vi "test Script CD with Configuration.vi"(8 "error in":errorcluster, 11 "TestCase in":refnum<class "Scripting.lvclass">) -> (0 "error out":errorcluster, 3 "TestCase out":refnum<class "Scripting.lvclass">)   [LabVIEW 2020, in "Scripting.lvclass"]
uses:
  Scripting.lvclass
  C:/Git/niveristand-custom-device-testing-tools/VeriStandScriptingTestCase/VeriStandScriptingTestCase.lvclass
  Shared/1553 Channel.ctl
  Shared/Address.ctl
  Shared/Message Definition.ctl
  Shared/Message Type.ctl
  Shared/Terminal Endpoint.ctl
  Shared/Parameter Definition.ctl
  niveristand-custom-device-testing-tools/VeriStandScriptingTestCase/VeriStandScriptingTestCase.lvclass/VeriStandScriptingTestCase.ctl
  niveristand-custom-device-testing-tools/VeriStandScriptingTestCase/Read Target.vi
  NationalInstruments.VeriStand.SystemDefinitionAPI
  <vilib>/addons/_JKI Toolkits/VI Tester/TestCase.llb/TestCase.lvclass
  Scripting/Ballard MIL-STD-1553 Scripting.lvlib
  C:/Program Files (x86)/National Instruments/LabVIEW 2020/vi.lib/addons/_JKI Toolkits/VI Tester/TestCase.llb/TestCase.lvclass
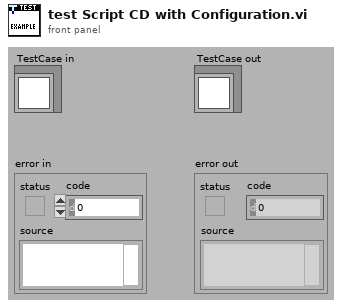
[diagram p1: front panel]
types:
  T1 = typedef "1553 Channel.ctl" = cluster{"HW channel":u16, "terminal addresses":T2[], "acyclic frame names":string[], "messages":T3[]}
  T2 = typedef "Address.ctl" = u16
  T3 = typedef "Message Definition.ctl" = cluster{"name":string, "message type":T4, "endpoint Tx":T5, "endpoint Rx":T5, "create timestamp channel":bool, "mode code":u16, "number of words":u16, "parameters":cluster{"name":string, "default value":dbl, "unit":string, "parameter definition":T6}[]}
  T4 = typedef "Message Type.ctl" = string
  T5 = typedef "Terminal Endpoint.ctl" = cluster{"terminal address":T2, "subaddress":T2}
  T6 = typedef "Parameter Definition.ctl" = cluster{"start index":i32, "size (bits)":i32, "encoding":enum16{"BNR", "BCD", "Discrete"}, "signed":bool, "multiplier":dbl, "offset":dbl}
  T7 = typedef "Custom Device API.lvlib/Custom Device Item Ref.ctl" = u64
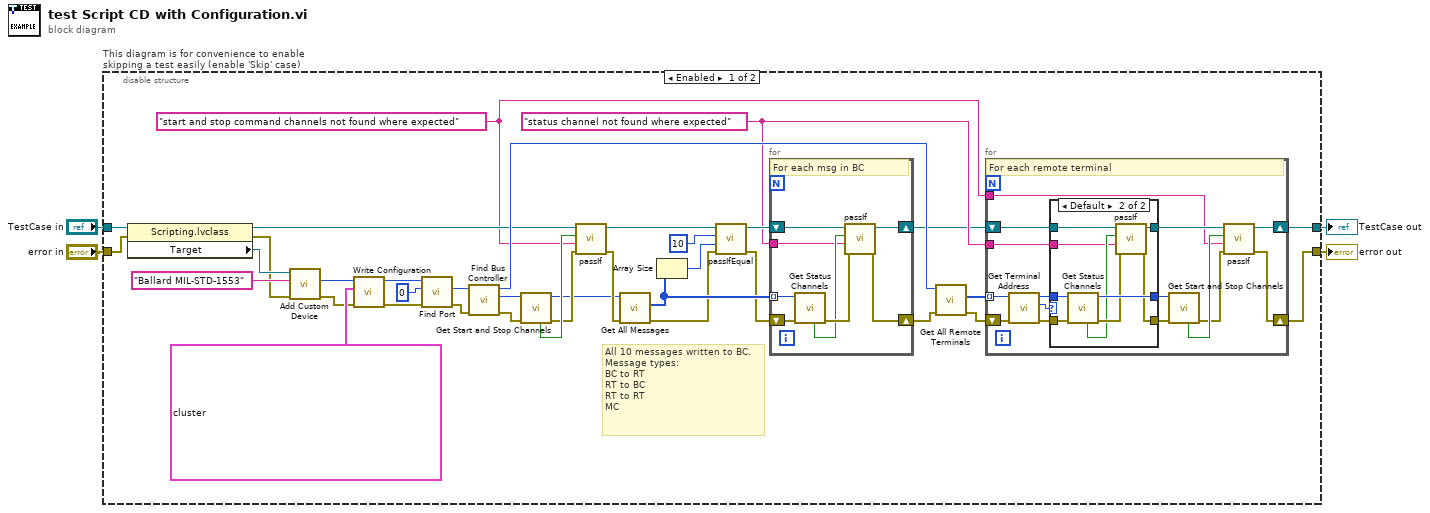
[diagram p0: block diagram]
diagram:
  n1 = disable-structure "This diagram is for convenience to enable skipping a test easily (enable 'Skip' case)" shown="Enabled" {
    disable-tunnel: "TestCase in" -> [w39 w79]
    disable-tunnel: [w22 w77] -> w1
    disable-tunnel: [w21 w78] -> w3
    disable-tunnel: "error in" -> [w34 w76]
    frame Enabled {
      w7 = "start and stop command channels not found where expected" ("name")
      w15 = "status channel not found where expected" ("name")
      # "All 10 messages written to BC.\nMessage types:\nBC to RT\nRT to BC\nRT to RT\nMC"
      n2 = property class="Scripting.lvclass"(reference=w39, error in=w34) -> (reference out=w11:refnum<class "Scripting.lvclass">, error out=w33:errorcluster, "Target"=w38:refnum<k24>)
      n3 = call "Add Custom Device.vi"("error in"=w33, "name"="Ballard MIL-STD-1553", "target in"=w38) -> ("error out"=w35:errorcluster, "Ballard MIL-STD 1553 custom device"=w37:T7)  [unwired: 6 in, 1 out]
      n4 = call "Write Configuration.vi"("error in"=w35, "1553 channels"=T1[] [{"HW channel"=0, "terminal addresses"=[0, 1, 15, 21, 31], "acyclic frame names"=["acyclicFrame ID56"], "messages"=[{"name"="BC to RT 1.2", "message type"="BC to RT", "endpoint Tx"={"terminal address"=0, "subaddress"=0}, "endpoint Rx"={"terminal address"=1, "subaddress"=2}, "create timestamp channel"=FALSE, "mode code"=0, "number of words"=3, "parameters"=[]}, {"name"="RT 31.15 to RT 21.21", "message type"="RT to RT", "endpoint Tx"={"terminal address"=15, "subaddress"=21}, "endpoint Rx"={"terminal address"=31, "subaddress"=21}, "create timestamp channel"=FALSE, "mode code"=0, "number of words"=11, "parameters"=[]}, {"name"="BC to RT 1.3", "message type"="BC to RT", "endpoint Tx"={"terminal address"=0, "subaddress"=0}, "endpoint Rx"={"terminal address"=1, "subaddress"=3}, "create timestamp channel"=FALSE, "mode code"=0, "number of words"=4, "parameters"=[]}, {"name"="RT 1.5 to BC", "message type"="RT to BC", "endpoint Tx"={"terminal address"=1, "subaddress"=5}, "endpoint Rx"={"terminal address"=0, "subaddress"=0}, "create timestamp channel"=FALSE, "mode code"=0, "number of words"=6, "parameters"=[]}, {"name"="RT 1.6 to BC", "message type"="RT to BC", "endpoint Tx"={"terminal address"=1, "subaddress"=6}, "endpoint Rx"={"terminal address"=0, "subaddress"=0}, "create timestamp channel"=FALSE, "mode code"=0, "number of words"=2, "parameters"=[]}, {"name"="RT 1.20 to RT 15.20", "message type"="RT to RT", "endpoint Tx"={"terminal address"=1, "subaddress"=20}, "endpoint Rx"={"terminal address"=15, "subaddress"=20}, "create timestamp channel"=FALSE, "mode code"=0, "number of words"=4, "parameters"=[]}, {"name"="MC 16", "message type"="MC", "endpoint Tx"={"terminal address"=1, "subaddress"=31}, "endpoint Rx"={"terminal address"=0, "subaddress"=0}, "create timestamp channel"=FALSE, "mode code"=16, "number of words"=1, "parameters"=[]}, {"name"="MC 17", "message type"="MC", "endpoint Tx"={"terminal address"=0, "subaddress"=0}, "endpoint Rx"={"terminal address"=1, "subaddress"=31}, "create timestamp channel"=FALSE, "mode code"=17, "number of words"=1, "parameters"=[]}, {"name"="BC to RT 31.28", "message type"="BC to RT", "endpoint Tx"={"terminal address"=0, "subaddress"=0}, "endpoint Rx"={"terminal address"=31, "subaddress"=28}, "create timestamp channel"=FALSE, "mode code"=0, "number of words"=6, "parameters"=[]}, {"name"="MC 1", "message type"="MC", "endpoint Tx"={"terminal address"=0, "subaddress"=0}, "endpoint Rx"={"terminal address"=31, "subaddress"=31}, "create timestamp channel"=FALSE, "mode code"=1, "number of words"=0, "parameters"=[]}]}], "Ballard MIL-STD 1553 custom device in"=w37) -> ("error out"=w28:errorcluster, "Ballard MIL-STD 1553 custom device out"=w30:T7)  [unwired: 7 in]
      n5 = call "Find Port.vi"("error in"=w28, "port number"=u16 0, "Ballard MIL-STD 1553 custom device in"=w30) -> ("error out"=w27:errorcluster, "port"=w26:T7)  [unwired: 5 in, 2 out]
      n6 = call "Find Bus Controller.vi"("error in"=w27, "port in"=w26) -> ("error out"=w9:errorcluster, "bus controller"=w6:T7, "port out"=w25:T7)  [unwired: 6 in, 1 out]
      n7 = call "Get Start and Stop Channels.vi"("error in"=w9, "terminal in"=w6) -> ("error out"=w12:errorcluster, "terminal out"=w5:T7, "found?"=w13:bool)  [unwired: 5 in, 2 out]
      n8 = call-dynamic "passIf.vi"("error in (no error)"=w12, "message (\"\")"=w7, "pass"=w13, "TestCase in"=w11) -> ("error out"=w8:errorcluster, "TestCase out"=w10:refnum<class "Scripting.lvclass">)  [unwired: 6 in]
      n9 = call "Get All Messages.vi"("error in"=w8, "port in"=w5) -> ("error out"=w19:errorcluster, "messages"=w20:T7[])  [unwired: 7 in, 1 out]
      n10 = Array Size(array=w20) -> (size(s)=w32:i32)
      n11 = call-dynamic "passIfEqual.vi"("error in (no error)"=w19, "y"=w32, "x"=10 ("size(s)"), "TestCase in"=w10) -> ("error out"=w18:errorcluster, "TestCase out"=w17:refnum<class "Scripting.lvclass">)  [unwired: 6 in]
      n12 = for {
        tunnel: w20 -> [w47] mode=indexing
        shift-right: [w43] -> w16
        shift-left: w18 -> [w48]
        shift-right: [w45] -> w14
        shift-left: w17 -> [w46]
        tunnel: w15 -> [w41]
        # "For each msg in BC"
        n13 = call "Get Status Channels.vi"("error in"=w48, "section reference in"=w47) -> ("error out"=w44:errorcluster, "found?"=w42:bool)  [unwired: 6 in, 2 out]
        n14 = call-dynamic "passIf.vi"("error in (no error)"=w44, "message (\"\")"=w41, "pass"=w42, "TestCase in"=w46) -> ("error out"=w43:errorcluster, "TestCase out"=w45:refnum<class "Scripting.lvclass">)  [unwired: 6 in]
      }
      n15 = call "Get All Remote Terminals.vi"("error in"=w16, "port in"=w25) -> ("error out"=w23:errorcluster, "remote terminals"=w24:T7[])  [unwired: 7 in, 1 out]
      n16 = for {
        tunnel: w24 -> [w52] mode=indexing
        shift-right: [w60] -> w21
        shift-left: w23 -> [w54]
        shift-right: [w62] -> w22
        shift-left: w14 -> [w58]
        tunnel: w15 -> [w55]
        tunnel: w7 -> [w49]
        # "For each remote terminal"
        n17 = call "Get Terminal Address.vi"("error in"=w54, "remote terminal in"=w52) -> ("error out"=w51:errorcluster, "terminal address"=w50:T2, "remote terminal out"=w53:T7)  [unwired: 6 in, 1 out]
        n18 = case shown="Default" w50 {
          tunnel: [w64 w75] -> w59
          tunnel: w58 -> [w66 w74]
          tunnel: [w66 w73] -> w57
          tunnel: [w65 w71] -> w56
          tunnel: w55 -> [_ w69]
          tunnel: w53 -> [w64 w68]
          tunnel: w51 -> [w65 w67]
          frame 31 {
          }
          frame Default {
            n19 = call "Get Status Channels.vi"("error in"=w67, "section reference in"=w68) -> ("error out"=w72:errorcluster, "section reference out"=w75:T7, "found?"=w70:bool)  [unwired: 6 in, 1 out]
            n20 = call-dynamic "passIf.vi"("error in (no error)"=w72, "message (\"\")"=w69, "pass"=w70, "TestCase in"=w74) -> ("error out"=w71:errorcluster, "TestCase out"=w73:refnum<class "Scripting.lvclass">)  [unwired: 6 in]
          }
        }
        n21 = call "Get Start and Stop Channels.vi"("error in"=w56, "terminal in"=w59) -> ("error out"=w61:errorcluster, "found?"=w63:bool)  [unwired: 5 in, 3 out]
        n22 = call-dynamic "passIf.vi"("error in (no error)"=w61, "message (\"\")"=w49, "pass"=w63, "TestCase in"=w57) -> ("error out"=w60:errorcluster, "TestCase out"=w62:refnum<class "Scripting.lvclass">)  [unwired: 6 in]
      }
    }
    frame Disabled {
      # "skip test result while test is under development"
      n23 = call <vilib>:"skip.vi"("error in (no error)"=w76, "TestCase in"=w79) -> ("error out"=w78:errorcluster, "TestCase out"=w77:refnum<class "Scripting.lvclass">)  [unwired: 8 in]
    }
  }
  "error out" <- w3
  "TestCase out" <- w1
